vi "DriveDiffGlobals.vi"() -> ()   [LabVIEW 2025]
panel:
  out "LeftSpeedTargFtPerSec":dbl
  out "RightSpeedTargFtPerSec":dbl
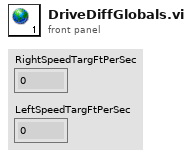
[diagram p1: front panel]
diagram:
